vi "Init.vi"(8 "error in":errorcluster) -> (0 "error out":errorcluster)   [LabVIEW 2018, in "Inputs.lvlib"]
doc: "This subVI enqueues the named action in to the communications queue along with the input data."
uses:
  Inputs.lvlib
  Private Controls/Module Data.ctl
  Private Controls/Module Action.ctl
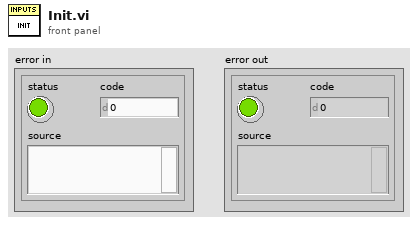
[diagram p1: front panel]
types:
  T1 = typedef "Inputs.lvlib/Module Data.ctl" = cluster{"Data":variant, "Action":T2}
  T2 = typedef "Inputs.lvlib/Module Action.ctl" = enum16{"Init", "RPMs", "Temps", "AI", "Timeout", "Error"}
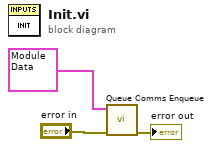
[diagram p0: block diagram]
diagram:
  n1 = call "Queue Comms Enqueue.vi"("error in (no error)"="error in", "element"=T1 {"Data"=variant, "Action"=enum."Init"}) -> ("error out"=→"error out":errorcluster)  [unwired: 9 in]
